vi "Power ON_OFF.vi"(8 "error in (no error)":errorcluster, 10 "Power":bool, 11 "SR3XXX HVPS in":refnum<class "SR3XXX HVPS.lvclass">) -> (0 "error out":errorcluster, 3 "SR3XXX HVPS out":refnum<class "SR3XXX HVPS.lvclass">)   [LabVIEW 2014, in "SR3XXX HVPS.lvclass"]
uses:
  SR3XXX HVPS.lvclass
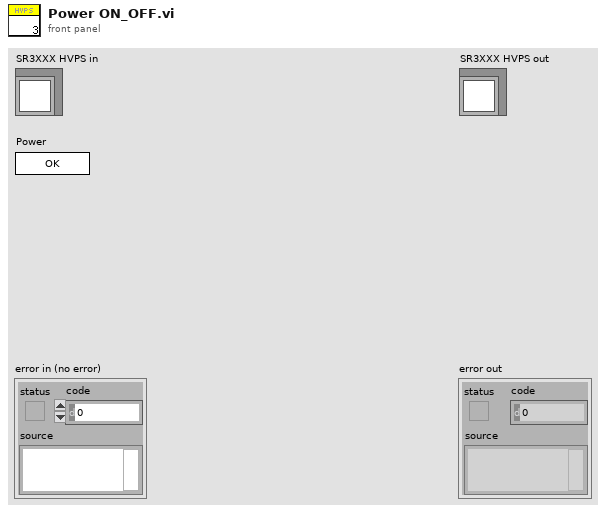
[diagram p1: front panel]
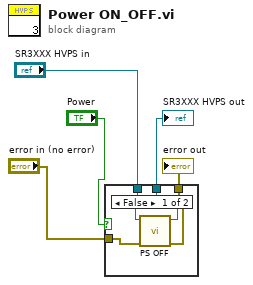
[diagram p0: block diagram]
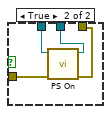
[diagram p2: hidden frame]
diagram:
  n1 = case shown="False" "Power" {
    tunnel: "SR3XXX HVPS in" -> [w9 w13]
    tunnel: [w8 w12] -> w4
    tunnel: "error in (no error)" -> [w6 w11]
    tunnel: [w7 w10] -> w2
    frame False {
      n2 = call "PS OFF.vi"("error in"=w6, "SR3XXX in"=w9) -> ("error out"=w7:errorcluster, "SR3XXX out"=w8:refnum<class "SR3XXX HVPS.lvclass">)  [unwired: 8 in]
    }
    frame True {
      n3 = call "PS On.vi"("error in"=w11, "SR3XXX in"=w13) -> ("error out"=w10:errorcluster, "SR3XXX out"=w12:refnum<class "SR3XXX HVPS.lvclass">)  [unwired: 8 in]
    }
  }
  "error out" <- w2
  "SR3XXX HVPS out" <- w4
